vi "EnumerateProperties.vi"(11 "TestManagerMsg.Test in":refnum<class "TestManagerMsg.Test.lvclass">) -> (2 "properties":string[](array[string]), 3 "TestManagerMsg.Test out":refnum<class "TestManagerMsg.Test.lvclass">)   [LabVIEW 2013, in "Caraya.lvlib" / "TestManagerMsg.Test.lvclass"]
uses:
  TestManagerMsg.Test.lvclass
  TestManagerMsg.Test.lvclass/TestManagerMsg.Test.ctl
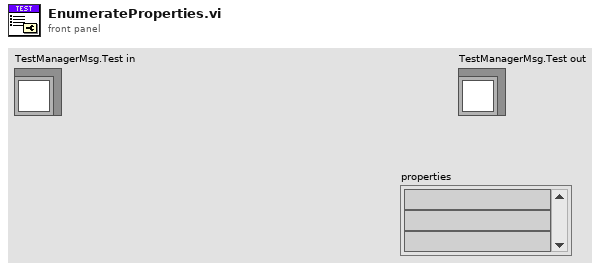
[diagram p1: front panel]
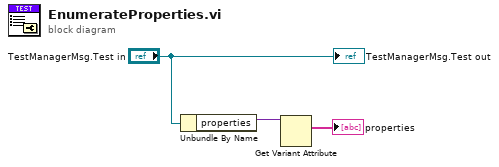
[diagram p0: block diagram]
diagram:
  n1 = Unbundle By Name("TestManagerMsg.Test in") -> ("properties"=w2:variant)
  n2 = Get Variant Attribute(Variant=w2) -> (names=→"properties":string[])  [unwired: 3 in, 3 out]
  "TestManagerMsg.Test out" <- "TestManagerMsg.Test in"
